vi "Teleop.vi"(10 "Match Info":T2={"Autonomous Elapsed Seconds"=0.0, "TeleOp Elapsed Seconds"=0.0, "Disabled Elapsed Seconds"=0.0, "Visited Autonomous"=FALSE, "Visited TeleOp"=FALSE, "Visited Disabled"=FALSE, "Autonomous Settings"={"Autonomous Style"=enum."Independent", "VI Refnum"=refnum}}, 11 "Call Context":T3) -> ()   [LabVIEW 2020]
doc: "This VI is called for each enabled TeleOp packet received from the DS. It is typically used to read from joysticks and other inputs and update I/O or setpoints for timed control loops. It should complete and return within 20 milliseconds or risk missing DS packets."
uses:
  <vilib>/Rock Robotics/WPI/DriverStation/WPI_DriverStationDerivedRobotMode.ctl
  <vilib>/Rock Robotics/WPI/DriverStation/WPI_DriverStationMatch Info.ctl
  <vilib>/Rock Robotics/WPI/Utilities/WPI_GetSetVariantRefNum.vi
  <vilib>/Rock Robotics/Network Tables/NT Write Boolean Array.vi
  <vilib>/Rock Robotics/Network Tables/NT Write Numeric Array.vi
panel:
  out "YRPHfH":T1
  in  "invert wheel":bool
  in  "invert throttle":bool
  in  "wheel":i32=4
  in  "throttle":i32=1
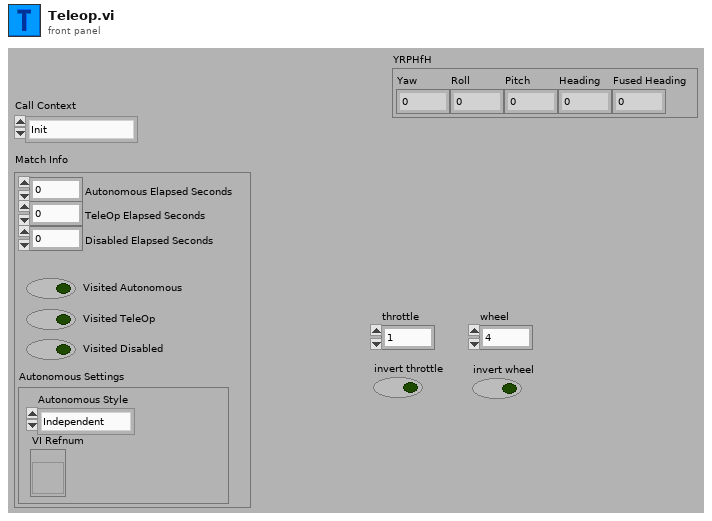
[diagram p1: front panel]
types:
  T1 = cluster{"Yaw":dbl, "Roll":dbl, "Pitch":dbl, "Heading":dbl, "Fused Heading":dbl}
  T2 = typedef "WPI_DriverStationMatch Info.ctl" = cluster{"Autonomous Elapsed Seconds":dbl, "TeleOp Elapsed Seconds":dbl, "Disabled Elapsed Seconds":dbl, "Visited Autonomous":bool, "Visited TeleOp":bool, "Visited Disabled":bool, "Autonomous Settings":cluster{"Autonomous Style":enum16{"Iterative", "Independent"}, "VI Refnum":refnum<vi>}}
  T3 = typedef "WPI_DriverStationDerivedRobotMode.ctl" = enum16{"Init", "Execute", "Stop"}
  T4 = typedef "WPI_JoystickDevRef.ctl" = cluster{"Device":T5}
  T5 = typedef "WPI_JoystickDeviceEnum.ctl" = enum16{"USB 0", "USB 1", "USB 2", "USB 3", "USB 4", "USB 5"}
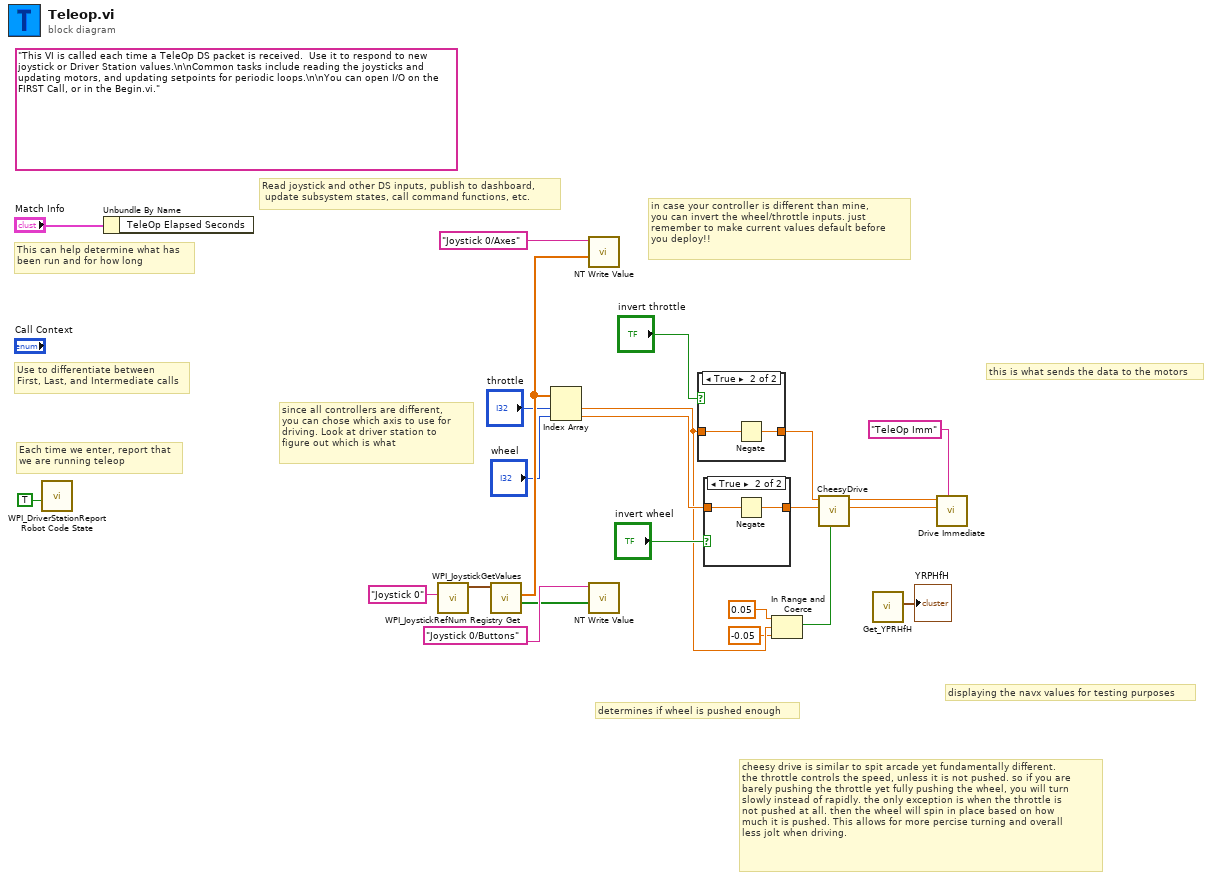
[diagram p0: block diagram]
diagram:
  (unwired) "This VI is called each time a TeleOp DS packet is received.  Use it to respond to new joystick or Driver Station values.\n\nCommon tasks include reading the joysticks and updating motors, and updating setpoints for periodic loops.\n\nYou can open I/O on the FIRST Call, or in the Begin.vi."
  # "determines if wheel is pushed enough"
  # "since all controllers are different,\nyou can chose which axis to use for \ndriving. Look at driver station to \nfigure out which is what"
  # "cheesy drive is similar to spit arcade yet fundamentally different. \nthe throttle controls the speed, unless it is not pushed. so if you are\nbarely pushing the throttle yet fully pushing the wheel, you will turn\nslowly instead of rapidly. the only exception is when the throttle is \nnot pushed at all. then the wheel will spin in place based on how\nmuch it is pushed. This allows for more percise turning and overall \nless jolt when driving."
  # "displaying the navx values for testing purposes"
  # "this is what sends the data to the motors"
  # "in case your controller is different than mine,\nyou can invert the wheel/throttle inputs. just\nremember to make current values default before \nyou deploy!!"
  # "Read joystick and other DS inputs, publish to dashboard,\n update subsystem states, call command functions, etc."
  # "Each time we enter, report that\nwe are running teleop"
  # "Use to differentiate between\nFirst, Last, and Intermediate calls"
  # "This can help determine what has\nbeen run and for how long"
  n1 = call <vilib>:"WPI_DriverStationReport Robot Code State.vi"("TeleOp"=TRUE ("Autonomous")) -> ()  [unwired: 10 in, 1 out]
  n2 = Unbundle By Name("Match Info") -> ()  [unwired: 1 out]
  n3 = call <vilib>:"WPI_JoystickRefNum Registry Get.vi"("refnum name"="Joystick 0") -> ("JoystickDevRef"=w20:T4)  [unwired: 1 in, 9 out]
  n4 = call <vilib>:"WPI_JoystickGetValues.vi"("JoystickDevRef"=w20) -> ("Buttons"=w15:bool[], "Axes"=w17:dbl[])  [unwired: 6 in, 3 out]
  n5 = Index Array(array=w17, index #1="throttle", index #2="wheel") -> (element #1=w3:dbl, element #2=w5:dbl)
  n6 = call-poly <vilib>:"NT Write Value.vi"("value"=w17, "name"="Joystick 0/Axes" ("Name")) -> ()  [unwired: 9 in, 1 out]
  n7 = call-poly <vilib>:"NT Write Value.vi"("value"=w15, "name"="Joystick 0/Buttons" ("Name")) -> ()  [unwired: 9 in, 1 out]
  n8 = case shown="True" "invert throttle" {
    tunnel: w3 -> [w24 w25]
    tunnel: [w24 w26] -> w10
    frame False {
    }
    frame True {
      n9 = Negate(x=w25) -> (-x=w26:dbl)
    }
  }
  n10 = case shown="True" "invert wheel" {
    tunnel: w5 -> [w27 w28]
    tunnel: [w27 w29] -> w9
    frame False {
    }
    frame True {
      n11 = Negate(x=w28) -> (-x=w29:dbl)
    }
  }
  n12 = In Range and Coerce(upper limit=0.05, x=w3, lower limit=-0.05 ("element")) -> (In Range?=w4:bool)  [unwired: 1 out]
  n13 = call "CheesyDrive.vi"("Quickturn"=w4, "Wheel"=w9, "Throttle"=w10) -> ("Right PWM"=w7:dbl, "Left PWM"=w8:dbl)  [unwired: 7 in]
  n14 = call <vilib>:"Get_YPRHfH.vi"() -> ("YRPHfH"=→"YRPHfH":T1)  [unwired: 11 in]
  n15 = call "Drive Immediate.vi"("Description"="TeleOp Imm", "Right Setpoint"=w7, "Left Setpoint"=w8) -> ()  [unwired: 8 in, 1 out]
